vi "Capture image.vi"(8 "error in (no error)":errorcluster, 9 "image metadata":T1={"title"="", "description"="", "ID"="", "version"="", "component type"=5} caption="Image metadata" {"component type" items=["standard", "hidden", "system", "unknown", "startup", "image"]}, 10 "destination file":path caption="Destination file", 11 "RT Management in":refnum<class "RT Management.lvclass">) -> (0 "error out":errorcluster, 3 "RT Management out":refnum<class "RT Management.lvclass">)   [LabVIEW 2015, in "RT Management.lvlib" / "RT Management.lvclass"]
doc: "Captures an image of an RT target and places the image at the path given in destination file."
uses:
  RT Management.lvclass
  <vilib>/nisyscfg/Software 1.2.ctl
  <vilib>/nisyscfg/Component Type.ctl
  RT Management.lvclass/RT Management.ctl
  Get SysCfg Session.vi
  <vilib>/nisyscfg/Create System Image (File).vi
  <vilib>/nisyscfg/nisyscfg.lvlib
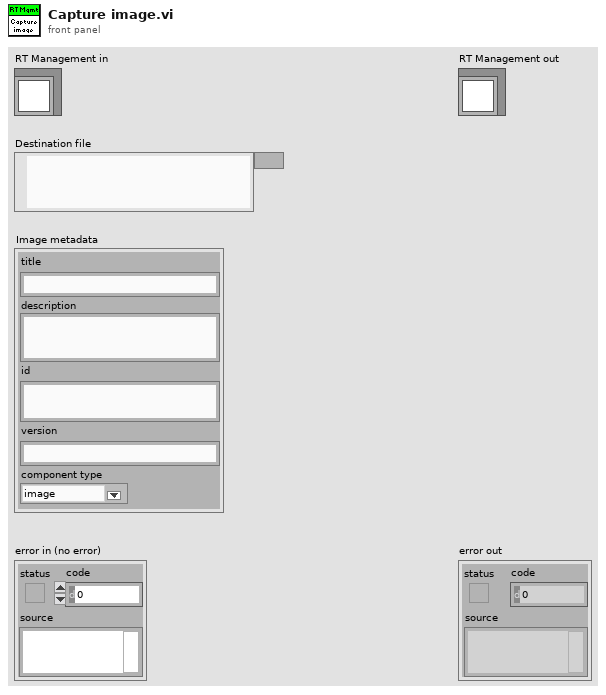
[diagram p1: front panel]
types:
  T1 = typedef "nisyscfg.lvlib/Software 1.2.ctl" = cluster{"title":string, "description":string, "ID":string, "version":string, "component type":T2}
  T2 = typedef "nisyscfg.lvlib/Component Type.ctl" = u32
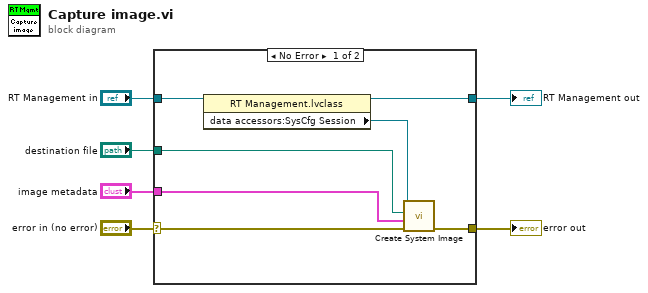
[diagram p0: block diagram]
diagram:
  n1 = case shown="No Error" "error in (no error)" {
    selector: "error in (no error)" -> [w12 w15]
    tunnel: [w11 w15] -> w5
    tunnel: [w7 w14] -> w3
    tunnel: "RT Management in" -> [w13 w14]
    tunnel: "destination file" -> [w9 _]
    tunnel: "image metadata" -> [w8 _]
    frame No Error {
      n2 = property class="RT Management.lvclass"(reference=w13) -> (reference out=w7:refnum<class "RT Management.lvclass">, "data accessors:SysCfg Session"=w10:refnum<k21>)  [unwired: 1 in, 1 out]
      n3 = call-poly <vilib>:"Create System Image.vi"("error in (no error)"=w12, "Image Metadata in"=w8, "Destination File"=w9, "Session in"=w10) -> ("error out"=w11:errorcluster)  [unwired: 5 in, 2 out]
    }
    frame Error {
    }
  }
  "error out" <- w5
  "RT Management out" <- w3
